vi "From Path Tree Data.vi"(11 "Tree Data":refnum<class "Tree Data.lvclass">) -> (2 "Path":path)   [LabVIEW 2017, in "Tree API.lvlib" / "Path.lvclass"]
doc: "Extract a Path value from Tree Data type."
uses:
  Path.lvclass
  Tree Data/Tree Data.lvclass
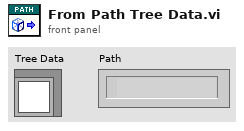
[diagram p1: front panel]
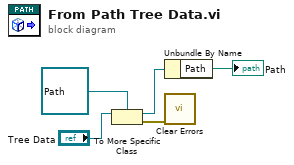
[diagram p0: block diagram]
diagram:
  n1 = To More Specific Class(target class=refnum<class "Path.lvclass"> refnum ("Path.lvclass"), reference="Tree Data") -> (specific class reference=w2:refnum<class "Path.lvclass">, error out=w1:errorcluster)  [unwired: 1 in]
  n2 = Unbundle By Name(w2) -> ("Path"=→"Path":path)
  n3 = call <vilib>:"Clear Errors.vi"("error in (no error)"=w1) -> ()  [unwired: 5 in, 2 out]
